vi "Safety_Check.vi"(1 "Adam Loop Count":i32, 2 "Ch Names":string[](array[string]), 3 "Values":dbl[](array[numeric]) format="%.2f") -> (0 "Scan comment":string)   [LabVIEW 2015]
uses:
  ADAM Client/Sub VIs/ADAM Controls/Update_scan_value.ctl
  Anemometry/Anemometry Sub Vis/Globals/Gas_management_global.vi
  ADAM_Global.vi
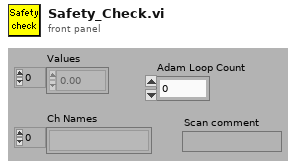
[diagram p1: front panel]
types:
  T1 = cluster{"Channel name":string, "Set value of A to":dbl, "Set value of B to":dbl, "Set value of C to":dbl, "Set value of D to":dbl}
  T2 = typedef "Update_scan_value.ctl" = cluster{"Channel Name":string, "New Value":dbl}
  T3 = enum16{"Append to Global", "Read Global then Clear"}
  T4 = enum16{"On", "Off", "Always On", "Always Off", "Delete"}
  T5 = typedef "LVDateTimeRec.ctl" = cluster{"fractional second":dbl, "second":i32, "minute":i32, "hour":i32, "day of month":i32, "month":i32, "year":i32, "day of week":i32, "day of year":i32, "DST":i32}
  T6 = cluster{"Channel name":string, "Set value of A to":dbl, "Set value of B to":dbl, "Set value of C to":dbl, "Set value of D to":dbl}[]
  T7 = typedef "Ch_description_ADAM.ctl" = cluster{"Ch Name":string, "Type":T8, "Function":T9, "Ch State":T10, "Calibration type":T11, "A":dbl, "B":dbl, "C":dbl, "D":dbl, "Comments":string, "Address":T12, "String":string, "Duty":u16}
  T8 = typedef "Module_type_ADAM.ctl" = string
  T9 = typedef "Function_ADAM.ctl" = enum16{"Analogue Input", "Digital Input", "Event counter", "Event rate", "Analogue Output", "Digital Output", "Relay Output"}
  T10 = typedef "Channel_State.ctl" = enum16{"On", "Off", "Always On", "Always Off"}
  T11 = typedef "Calib_type_ADAM.ctl" = enum16{"Raw", "Bx + A", "Cx^2 + Bx + A", "Dx^3 + Cx^2 + Bx + A", "In Band", "Hi-Tec Q", "Hi-Tec M_dot", "Text"}
  T12 = typedef "Address.ctl" = cluster{"Main":i32, "Ch.":i32, "Sub":i32, "Port Name":string}
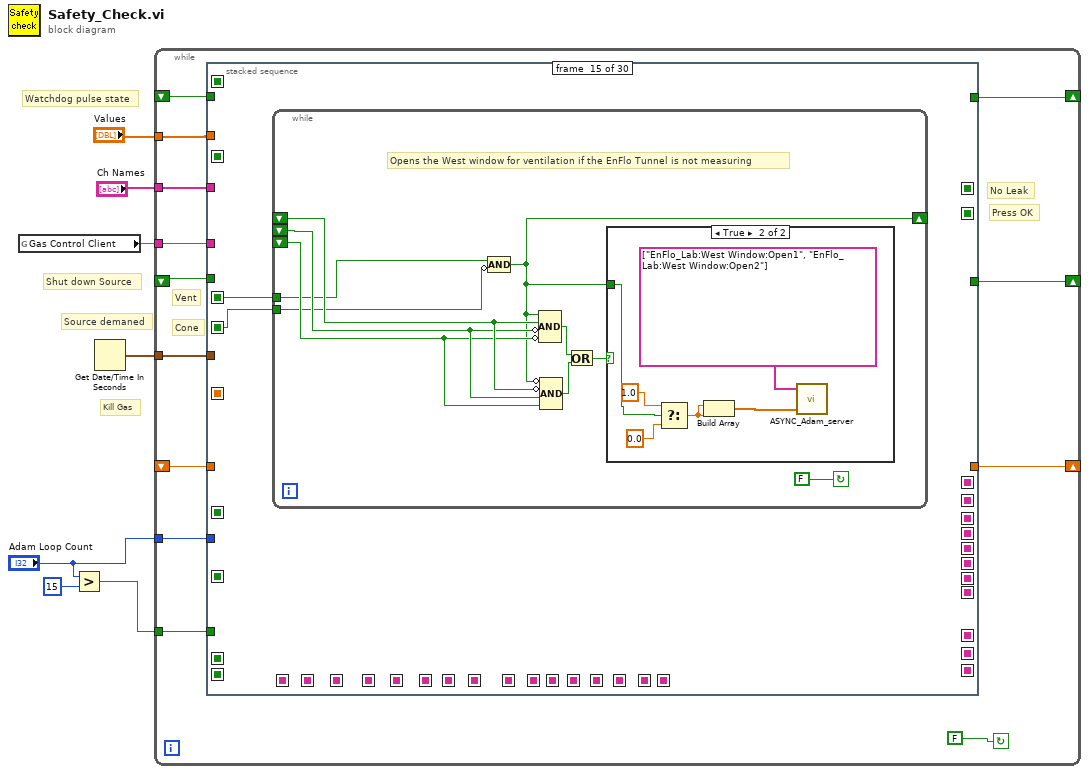
[diagram p0: block diagram]
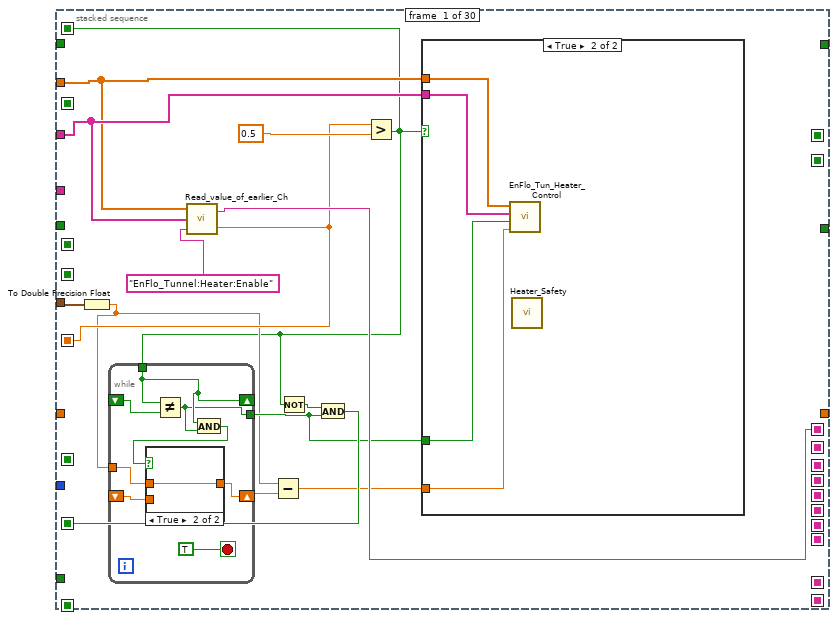
[diagram p2: hidden frame]
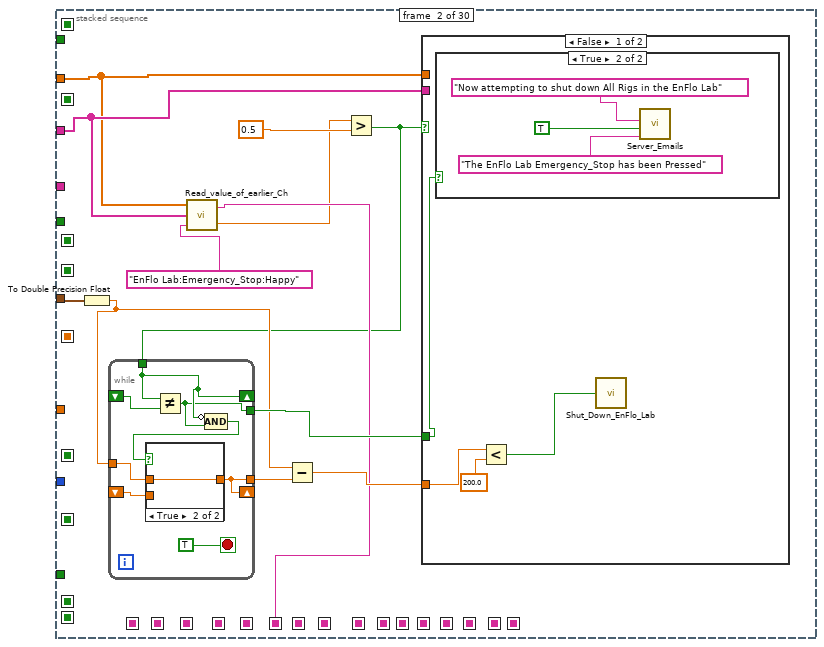
[diagram p5: hidden frame]
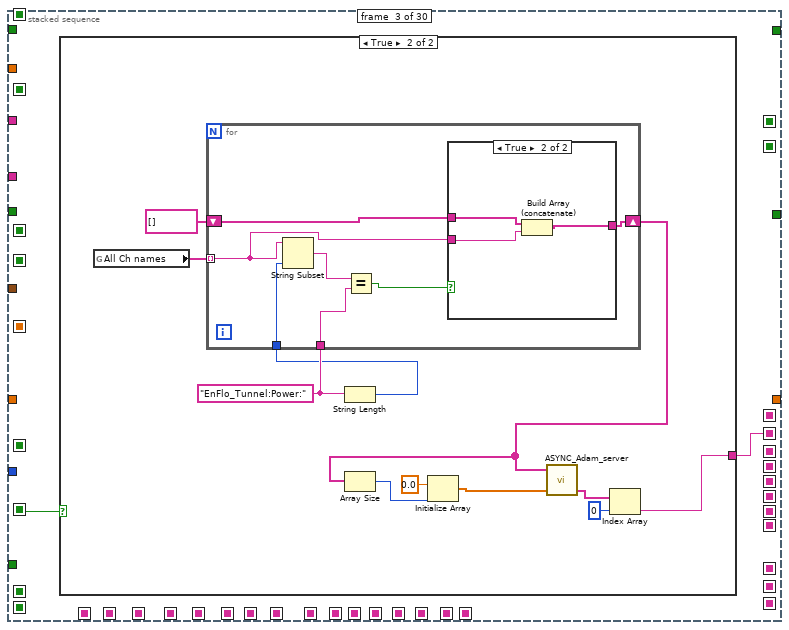
[diagram p9: hidden frame]
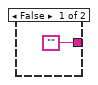
[diagram p10: hidden frame]
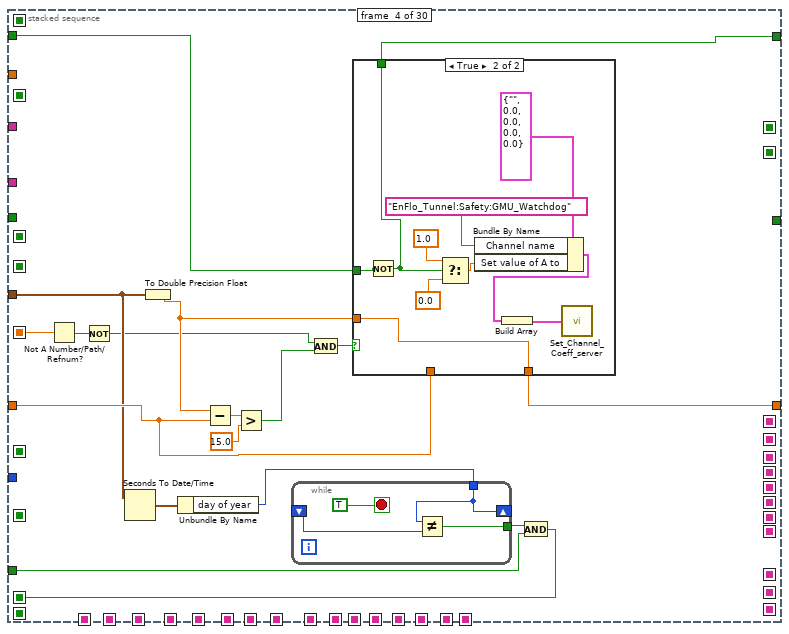
[diagram p12: hidden frame]
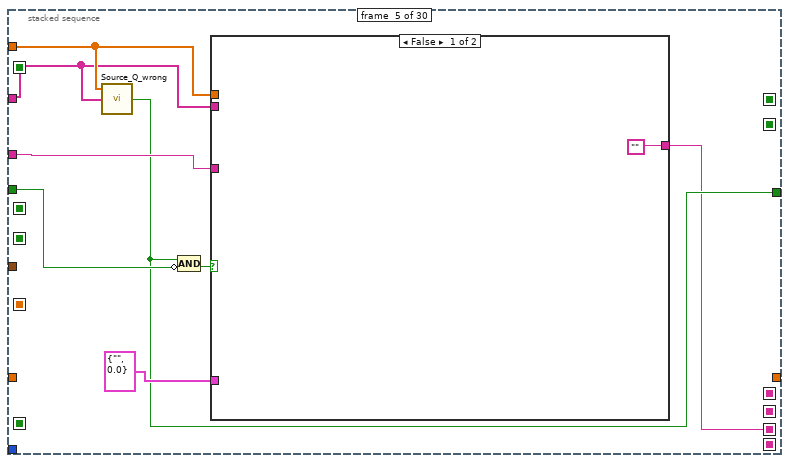
[diagram p14: hidden frame]
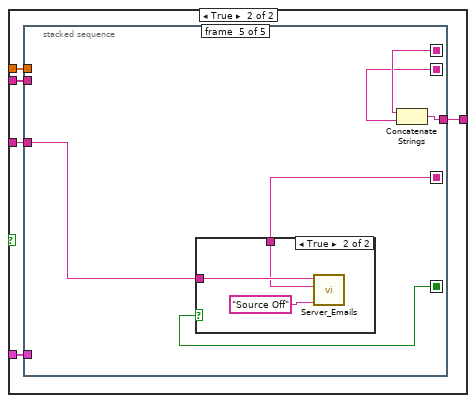
[diagram p15: hidden frame]
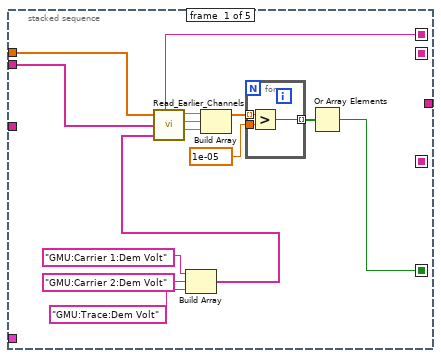
[diagram p16: hidden frame]
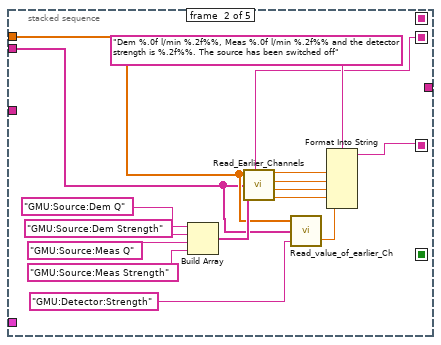
[diagram p17: hidden frame]
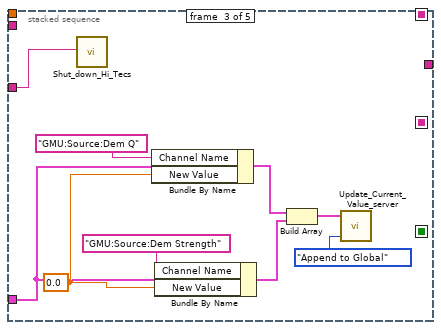
[diagram p18: hidden frame]
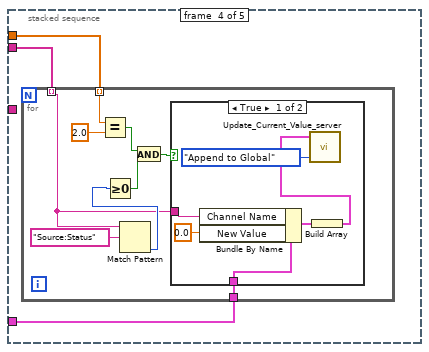
[diagram p19: hidden frame]
diagram:
  # "Shut down Source"
  # "Source demaned"
  # "Watchdog pulse state"
  # "Kill Gas"
  n1 = global read "Gas_management_global.vi" "Gas Control Client"() -> (w5:string)
  n2 = Greater?(x="Adam Loop Count", y=15) -> (0:w3:bool)
  n3 = Get Date/Time In Seconds() -> (seconds since 1Jan1904=w2:timestamp)
  n4 = while {
    shift-left: _ -> [w15]
    shift-right: [w14] -> _
    shift-left: _ -> [w17]
    shift-right: [w16] -> _
    tunnel: w5 -> [w19]
    tunnel: "Ch Names" -> [w20]
    tunnel: "Values" -> [w18]
    shift-right: [w12] -> _
    shift-left: _ -> [w11]
    tunnel: w3 -> [w10]
    tunnel: w2 -> [w9]
    tunnel: "Adam Loop Count" -> [w8]
    stop <- FALSE continue-if-true
    # "Cone"
    # "Vent"
    # "Press OK"
    # "No Leak"
    n5 = stacked-sequence {
      seq-local: [_ _ _ _ _ _ _ w260 _ _ _ _ _ _ _ _ _ _ _ _ _ _ _ _ _ _ _ _ _ _] -> [_ _ _ _ _ _ _ _ _ _ _ _ _ _ _ _ _ _ _ w623 _ _ _ _ _ _ _ _ _ _]
      seq-local: [w28 _ _ _ _ _ _ _ _ _ _ _ _ _ _ _ _ _ _ _ _ _ _ _ _ _ _ _ _ _] -> [_ _ w79 _ _ _ _ _ _ _ _ _ _ _ _ _ _ _ _ _ _ _ _ _ _ _ _ _ _ _]
      seq-local: [_ _ _ w109 _ _ _ _ _ _ _ _ _ _ _ _ _ _ _ _ _ _ _ _ _ _ _ _ _ _] -> [_ _ _ _ _ _ _ _ _ _ _ _ _ _ _ _ _ _ _ _ _ _ _ _ _ _ _ _ _ _]
      seq-local: [_ _ _ _ _ _ _ _ _ _ _ _ _ _ _ _ _ _ _ _ _ _ _ w753 _ _ _ _ _ _] -> [_ _ _ _ _ _ _ _ _ _ _ _ _ _ _ _ _ _ _ _ _ _ _ _ w765 _ _ _ _ _]
      seq-local: [_ _ _ _ _ _ _ _ _ _ _ _ _ _ _ _ _ _ _ _ _ _ _ _ w760 _ _ _ _ _] -> [_ _ _ _ _ _ _ _ _ _ _ _ _ _ _ _ _ _ _ _ _ _ _ _ _ _ _ w874 _ _]
      seq-local: [w30 _ _ _ _ _ _ _ _ _ _ _ _ _ _ _ _ _ _ _ _ _ _ _ _ _ _ _ _ _] -> [_ _ _ _ _ _ _ _ _ _ _ _ _ _ _ _ _ _ _ _ _ _ _ _ _ _ _ _ _ w957]
      seq-local: [_ _ w78 _ _ _ _ _ _ _ _ _ _ _ _ _ _ _ _ _ _ _ _ _ _ _ _ _ _ _] -> [_ _ _ _ _ _ _ _ _ _ _ _ _ _ _ _ _ _ _ _ _ _ _ _ _ _ _ _ _ w956]
      seq-local: [_ _ _ _ w137 _ _ _ _ _ _ _ _ _ _ _ _ _ _ _ _ _ _ _ _ _ _ _ _ _] -> [_ _ _ _ _ _ _ _ _ _ _ _ _ _ _ _ _ _ _ _ _ _ _ _ _ _ _ _ _ w955]
      seq-local: [_ _ _ _ _ w220 _ _ _ _ _ _ _ _ _ _ _ _ _ _ _ _ _ _ _ _ _ _ _ _] -> [_ _ _ _ _ _ _ _ _ _ _ _ _ _ _ _ _ _ _ _ _ _ _ _ _ _ _ _ _ w954]
      seq-local: [_ _ _ _ _ _ w240 _ _ _ _ _ _ _ _ _ _ _ _ _ _ _ _ _ _ _ _ _ _ _] -> [_ _ _ _ _ _ _ _ _ _ _ _ _ _ _ _ _ _ _ _ _ _ _ _ _ _ _ _ _ w953]
      seq-local: [_ _ _ _ _ _ _ w259 _ _ _ _ _ _ _ _ _ _ _ _ _ _ _ _ _ _ _ _ _ _] -> [_ _ _ _ _ _ _ _ _ _ _ _ _ _ _ _ _ _ _ _ _ _ _ _ _ _ _ _ _ w952]
      seq-local: [_ _ _ _ _ _ _ _ _ _ w371 _ _ _ _ _ _ _ _ _ _ _ _ _ _ _ _ _ _ _] -> [_ _ _ _ _ _ _ _ _ _ _ _ _ _ _ _ _ _ _ _ _ _ _ _ _ _ _ _ _ w951]
      seq-local: [_ _ _ _ _ _ _ _ _ _ _ w403 _ _ _ _ _ _ _ _ _ _ _ _ _ _ _ _ _ _] -> [_ _ _ _ _ _ _ _ _ _ _ _ _ _ _ _ _ _ _ _ _ _ _ _ _ _ _ _ _ w942]
      seq-local: [_ _ _ _ _ _ _ _ _ _ _ _ _ _ _ _ w549 _ _ _ _ _ _ _ _ _ _ _ _ _] -> [_ _ _ _ _ _ _ _ _ _ _ _ _ _ _ _ _ _ _ _ _ _ _ _ _ _ _ _ _ w941]
      seq-local: [_ _ _ _ _ _ _ _ _ _ _ _ _ _ _ _ _ _ _ w624 _ _ _ _ _ _ _ _ _ _] -> [_ _ _ _ _ _ _ _ _ _ _ _ _ _ _ _ _ _ _ _ _ _ _ _ _ _ _ _ _ w944]
      seq-local: [_ _ _ _ _ _ _ _ _ _ _ _ _ _ _ _ _ _ _ _ w652 _ _ _ _ _ _ _ _ _] -> [_ _ _ _ _ _ _ _ _ _ _ _ _ _ _ _ _ _ _ _ _ _ _ _ _ _ _ _ _ w945]
      seq-local: [_ _ _ _ _ _ _ _ _ _ _ _ _ _ _ _ _ _ _ _ _ _ _ w747 _ _ _ _ _ _] -> [_ _ _ _ _ _ _ _ _ _ _ _ _ _ _ _ _ _ _ _ _ _ _ _ _ _ _ _ _ w946]
      seq-local: [_ _ _ _ _ _ _ _ _ _ _ _ _ _ _ _ _ _ _ _ _ _ _ _ w757 _ _ _ _ _] -> [_ _ _ _ _ _ _ _ _ _ _ _ _ _ _ _ _ _ _ _ _ _ _ _ _ _ _ _ _ w947]
      seq-local: [_ _ _ _ _ _ _ _ _ _ _ _ w434 _ _ _ _ _ _ _ _ _ _ _ _ _ _ _ _ _] -> [_ _ _ _ _ _ _ _ _ _ _ _ _ _ _ _ _ _ _ _ _ _ _ _ _ _ _ _ _ w948]
      seq-local: [_ _ _ _ _ _ _ _ _ _ _ _ _ _ _ _ _ _ _ _ _ _ _ _ _ _ w836 _ _ _] -> [_ _ _ _ _ _ _ _ _ _ _ _ _ _ _ _ _ _ _ _ _ _ _ _ _ _ _ _ _ w949]
      seq-local: [_ _ _ _ _ _ _ _ _ _ _ _ _ _ _ _ _ _ _ _ _ _ _ _ _ _ _ w872 _ _] -> [_ _ _ _ _ _ _ _ _ _ _ _ _ _ _ _ _ _ _ _ _ _ _ _ _ _ _ _ _ w950]
      seq-local: [w29 _ _ _ _ _ _ _ _ _ _ _ _ _ _ _ _ _ _ _ _ _ _ _ _ _ _ _ _ _] -> [_ _ _ w107 _ _ _ _ _ _ _ _ _ _ _ _ _ _ _ _ _ _ _ _ _ _ _ _ _ _]
      seq-local: [_ _ _ _ _ _ _ _ w278 _ _ _ _ _ _ _ _ _ _ _ _ _ _ _ _ _ _ _ _ _] -> [_ _ _ _ _ _ _ _ _ _ _ _ _ _ _ _ _ _ _ w622 _ _ _ _ _ _ _ _ _ _]
      seq-local: [_ _ _ _ _ _ _ _ w277 _ _ _ _ _ _ _ _ _ _ _ _ _ _ _ _ _ _ _ _ _] -> [_ _ _ _ _ _ _ _ _ _ _ _ _ _ _ _ _ _ _ _ _ _ _ _ _ _ _ _ _ w940]
      seq-local: [_ _ _ _ _ _ _ _ w276 _ _ _ _ _ _ _ _ _ _ _ _ _ _ _ _ _ _ _ _ _] -> [_ _ _ _ _ _ _ _ _ w308 _ _ _ _ _ _ _ _ _ _ _ _ _ w748 w756 w821 _ _ _ _]
      seq-local: [_ _ _ _ _ _ _ _ _ w305 _ _ _ _ _ _ _ _ _ _ _ _ _ _ _ _ _ _ _ _] -> [_ _ _ _ _ _ _ _ _ _ _ _ _ _ _ _ _ _ _ _ _ _ _ _ _ _ _ _ _ w938]
      seq-local: [_ _ _ _ _ _ _ _ _ _ _ _ _ _ _ w503 _ _ _ _ _ _ _ _ _ _ _ _ _ _] -> [_ _ _ _ _ _ _ _ _ _ _ _ _ _ _ _ _ _ _ _ _ _ _ _ _ _ _ _ _ w939]
      seq-local: [_ _ _ _ _ _ _ _ _ _ _ _ _ _ _ _ _ _ _ _ _ _ w715 _ _ _ _ _ _ _] -> [_ _ _ _ _ _ _ _ _ _ _ _ _ _ _ _ _ _ _ _ _ _ _ _ _ _ _ _ _ w937]
      seq-local: [_ _ _ _ _ _ _ _ _ _ _ _ _ w462 _ _ _ _ _ _ _ _ _ _ _ _ _ _ _ _] -> [_ _ _ _ _ _ _ _ _ _ _ _ _ _ _ _ _ _ _ _ _ _ _ _ _ _ _ _ _ w936]
      seq-local: [_ w52 _ _ _ _ _ _ _ _ _ _ _ _ _ _ _ _ _ _ _ _ _ _ _ _ _ _ _ _] -> [_ _ _ _ _ _ _ _ _ _ _ _ _ _ _ _ _ _ _ _ _ _ _ _ _ _ _ _ _ w935]
      seq-local: [_ _ _ _ _ _ _ _ _ _ _ _ _ _ _ _ _ _ _ _ _ _ _ _ _ _ _ _ w894 _] -> [_ _ _ _ _ _ _ _ _ _ _ _ _ _ _ _ _ _ _ _ _ _ _ _ _ _ _ _ _ w934]
      seq-local: [_ _ _ _ _ _ _ _ _ _ _ _ _ _ _ _ _ w570 _ _ _ _ _ _ _ _ _ _ _ _] -> [_ _ _ _ _ _ _ _ _ _ _ _ _ _ _ _ _ _ _ _ _ _ _ _ _ _ _ _ _ w932]
      seq-local: [_ _ _ _ _ _ _ _ _ _ _ _ _ _ _ _ _ _ w602 _ _ _ _ _ _ _ _ _ _ _] -> [_ _ _ _ _ _ _ _ _ _ _ _ _ _ _ _ _ _ _ _ _ _ _ _ _ _ _ _ _ w933]
      seq-local: [w21 _ _ _ _ _ _ _ _ _ _ _ _ _ _ _ _ _ _ _ _ _ _ _ _ _ _ _ _ _] -> [_ _ _ _ _ _ _ _ _ _ _ _ _ _ _ _ _ _ _ _ w651 w672 _ _ _ _ _ _ _ _]
      seq-local: [_ _ _ _ _ _ _ _ _ _ _ _ _ _ _ _ _ _ _ _ _ w670 _ _ _ _ _ _ _ _] -> [_ _ _ _ _ _ _ _ _ _ _ _ _ _ _ _ _ _ _ _ _ _ _ _ _ _ _ _ _ w931]
      seq-local: [_ _ _ _ _ _ _ _ _ _ _ _ _ _ _ _ _ _ _ _ _ _ _ _ _ w820 _ _ _ _] -> [_ _ _ _ _ _ _ _ _ _ _ _ _ _ _ _ _ _ _ _ _ _ _ _ _ _ _ _ _ w930]
      seq-local: [_ _ _ _ _ _ _ _ _ _ _ _ w423 _ _ _ _ _ _ _ _ _ _ _ _ _ _ _ _ _] -> [_ _ _ _ _ _ _ _ _ _ _ _ _ _ w483 _ _ _ _ _ _ _ _ _ _ _ _ _ _ _]
      seq-local: [_ _ _ _ _ _ _ _ _ _ _ _ _ w461 _ _ _ _ _ _ _ _ _ _ _ _ _ _ _ _] -> [_ _ _ _ _ _ _ _ _ _ _ _ _ _ w484 _ _ _ _ _ _ _ _ _ _ _ _ _ _ _]
      tunnel: w20 -> [w32 w58 _ _ w139 w227 w242 w261 w279 w306 w372 w404 w433 w463 _ w504 w551 w572 w604 w625 w656 w676 w709 w751 w766 _ w839 _ _ _]
      tunnel: w19 -> [_ _ _ _ w144 _ w241 _ _ _ _ _ _ _ _ _ _ _ _ _ _ _ _ _ _ _ _ _ _ _]
      tunnel: w18 -> [w31 w57 _ _ w140 w223 w243 w262 w280 w307 w373 w405 w431 w464 _ w505 w552 w573 w605 w626 w657 w677 w708 w752 w767 _ w840 _ _ _]
      tunnel: w17 -> [_ _ _ w120 _ _ _ _ _ _ _ _ _ _ _ _ _ _ _ _ _ _ _ _ _ _ _ _ _ _]
      tunnel: [_ _ _ w119 _ _ _ _ _ _ _ _ _ _ _ _ _ _ _ _ _ _ _ _ _ _ _ _ _ _] -> w16
      tunnel: w15 -> [_ _ _ _ w143 _ _ _ _ _ _ _ _ _ _ _ _ _ _ _ _ _ _ _ _ _ _ _ _ _]
      tunnel: [_ _ _ _ w138 _ _ _ _ _ _ _ _ _ _ _ _ _ _ _ _ _ _ _ _ _ _ _ _ _] -> w14
      tunnel: [_ _ _ w118 _ _ _ _ _ _ _ _ _ _ _ _ _ _ _ _ _ _ _ _ _ _ _ _ _ _] -> w12
      tunnel: w11 -> [_ _ _ w114 _ _ _ _ _ _ _ _ _ _ _ _ _ _ _ _ _ _ _ _ _ _ _ _ _ _]
      tunnel: w10 -> [_ _ _ w110 _ _ _ _ _ _ _ _ w435 _ _ w501 w550 w571 w603 _ _ _ _ _ w761 w819 _ w873 _ _]
      tunnel: w9 -> [w25 w55 _ w108 _ _ _ _ _ _ _ _ _ _ _ w502 _ _ _ _ _ _ _ _ _ _ _ _ _ _]
      tunnel: w8 -> [_ _ _ _ _ _ _ _ _ _ _ _ _ _ _ _ _ _ _ _ _ _ _ _ _ _ _ _ w907 _]
      frame #0 {
        n6 = To Double Precision Float(number=w25) -> (double precision float=w24:dbl)
        n7 = call "Read_value_of_earlier_Ch.vi"("Desired Ch to Read"="EnFlo_Tunnel:Heater:Enable", "Ch names"=w32, "Present scan array"=w31) -> ("Value"=w29:dbl, "Scan comment"=w30:string)  [unwired: 1 in]
        n8 = Greater?(x=w29, y=0.5) -> (0:w21:bool)
        n9 = while {
          shift-right: [w40] -> _
          shift-left: _ -> [w42]
          tunnel: w21 -> [w40]
          tunnel: [w39] -> w26
          shift-right: [w37] -> w23
          shift-left: _ -> [w35]
          tunnel: w24 -> [w36]
          stop <- TRUE stop-if-true
          n10 = Not Equal?(x=w40, y=w42) -> (x != y?=w39:bool)
          n11 = And(x=w40, y=w39) -> (x .and. y?=w38:bool)
          n12 = case shown="True" w38 {
            tunnel: [w43 w44] -> w37
            tunnel: w36 -> [_ w44]
            tunnel: w35 -> [w43 _]
            frame False {
            }
            frame True {
            }
          }
        }
        n13 = Subtract(x=w24, y=w23) -> (x-y=w22:dbl)
        n14 = Not(x=w21) -> (.not. x?=w27:bool)
        n15 = And(x=w27, y=w26) -> (x .and. y?=w28:bool)
        n16 = case shown="True" w21 {
          tunnel: w31 -> [_ w48]
          tunnel: w32 -> [_ w47]
          tunnel: w26 -> [_ w46]
          tunnel: w22 -> [_ w45]
          frame False {
          }
          frame True {
            n17 = call "EnFlo_Tun_Heater_Control.vi"("Heaters Enabled time (s)"=w45, "Heaters Just Enabled"=w46, "Ch Names"=w47, "Values"=w48) -> ()  [unwired: 1 in]
            n18 = call "Heater_Safety.vi"() -> ()  [unwired: 3 in, 5 out]
          }
        }
      }
      frame #1 {
        n19 = To Double Precision Float(number=w55) -> (double precision float=w54:dbl)
        n20 = call "Read_value_of_earlier_Ch.vi"("Desired Ch to Read"="EnFlo Lab:Emergency_Stop:Happy", "Ch names"=w58, "Present scan array"=w57) -> ("Value"=w50:dbl, "Scan comment"=w52:string)  [unwired: 1 in]
        n21 = Greater?(x=w50, y=0.5) -> (0:w51:bool)
        n22 = while {
          shift-right: [w66] -> _
          shift-left: _ -> [w68]
          tunnel: w51 -> [w66]
          tunnel: [w65] -> w56
          shift-right: [w61] -> _
          shift-left: _ -> [w62]
          tunnel: w54 -> [w63]
          tunnel: [w61] -> w49
          stop <- TRUE stop-if-true
          n23 = Not Equal?(x=w66, y=w68) -> (x != y?=w65:bool)
          n24 = Compound Arithmetic op=AND(invert w66, w65) -> (w64:bool)
          n25 = case shown="True" w64 {
            tunnel: [w69 w70] -> w61
            tunnel: w63 -> [_ w70]
            tunnel: w62 -> [w69 _]
            frame False {
            }
            frame True {
            }
          }
        }
        n26 = Subtract(x=w54, y=w49) -> (x-y=w53:dbl)
        n27 = case shown="False" w51 {
          tunnel: w57 -> [_ _]
          tunnel: w58 -> [_ _]
          tunnel: w56 -> [w72 _]
          tunnel: w53 -> [w74 _]
          frame False {
            n28 = case shown="True" w72 {
              frame False {
              }
              frame True {
                n29 = call "Server_Emails.vi"("Message"="Now attempting to shut down All Rigs in the EnFlo Lab", "Contact All clients?"=TRUE, "Subject"="The EnFlo Lab Emergency_Stop has been Pressed") -> ()  [unwired: 2 in, 3 out]
              }
            }
            n30 = Less?(x=w74, y=200.0) -> (x < y?=w71:bool)
            n31 = call "Shut_Down_EnFlo_Lab.vi"("Initial Shutdown"=w71) -> ()
          }
          frame True {
          }
        }
      }
      frame #2 {
        n32 = case shown="True" w79 {
          tunnel: ["" w82] -> w78
          frame False {
          }
          frame True {
            w91 = "EnFlo_Tunnel:Power:"
            n33 = global read "ADAM_Global.vi" "All Ch names"() -> (w81:string[])
            n34 = String Length(string=w91) -> (length=w90:i32)
            n35 = for {
              shift-right: [w93] -> w86
              shift-left: string[] [] -> [w94]
              tunnel: w81 -> [w97] mode=indexing
              tunnel: w90 -> [w98]
              tunnel: w91 -> [w95]
              n36 = String Subset(string=w97, length (rest)=w98) -> (substring=w96:string)  [unwired: 1 out]
              n37 = Equal?(x=w96, y=w95) -> (x = y?=w92:bool)
              n38 = case shown="True" w92 {
                tunnel: w97 -> [_ w102]
                tunnel: w94 -> [w99 w100]
                tunnel: [w99 w101] -> w93
                frame False {
                }
                frame True {
                  n39 = Build Array (concatenate)(w100, w102) -> (w101:string[])
                }
              }
            }
            n40 = Array Size(array=w86) -> (size(s)=w87:i32)
            n41 = Initialize Array(0.0 ("element"), w87) -> (w85:dbl[])
            n42 = call "ASYNC_Adam_server.vi"("Values"=w85, "Channel Names"=w86) -> ("Scan Comments"=w84:string[])  [unwired: 1 in, 2 out]
            n43 = Index Array(array=w84, index=0) -> (element=w82:string)
          }
        }
      }
      frame #3 {
        n44 = Not A Number/Path/Refnum?(number/path/refnum=w107) -> (NaN/Path/Refnum?=w106:bool)
        n45 = Not(x=w106) -> (.not. x?=w104:bool)
        n46 = Seconds To Date/Time(time stamp (now)=w108) -> (date time rec=w113:T5)  [unwired: 1 in]
        n47 = To Double Precision Float(number=w108) -> (double precision float=w117:dbl)
        n48 = Unbundle By Name(w113) -> ("day of year"=w112:i32)
        n49 = Subtract(x=w117, y=w114) -> (x-y=w116:dbl)
        n50 = Greater?(x=w116, y=15.0) -> (0:w105:bool)
        n51 = while {
          shift-right: [w124] -> _
          shift-left: _ -> [w123]
          tunnel: w112 -> [w124]
          tunnel: [w122] -> w111
          stop <- TRUE stop-if-true
          n52 = Not Equal?(x=w124, y=w123) -> (x != y?=w122:bool)
        }
        n53 = And(x=w104, y=w105) -> (x .and. y?=w103:bool)
        n54 = case shown="True" w103 {
          tunnel: w120 -> [w125 w129]
          tunnel: [w125 w128] -> w119
          tunnel: [w126 w127] -> w118
          tunnel: w117 -> [_ w127]
          tunnel: w114 -> [w126 _]
          frame False {
          }
          frame True {
            n55 = Not(x=w129) -> (.not. x?=w128:bool)
            n56 = Select(t=1.0 ("Suction"), s=w128, f=0.0 ("Suction")) -> (s? t:f=w132:dbl)
            n57 = Bundle By Name(cluster=T1 {"Channel name"="", "Set value of A to"=0.0, "Set value of B to"=0.0, "Set value of C to"=0.0, "Set value of D to"=0.0}, "Channel name"="EnFlo_Tunnel:Safety:GMU_Watchdog" ("Desired Ch to Read"), "Set value of A to"=w132) -> (w136:T1)
            n58 = Build Array(w136) -> (w131:T6)
            n59 = call "Set_Channel_Coeff_server.vi"("Set Array"=w131) -> ()
          }
        }
        n60 = And(x=w111, y=w110) -> (x .and. y?=w109:bool)
      }
      frame #4 {
        n61 = call "Source_Q_wrong.vi"("Ch Names"=w139, "Values"=w140) -> ("Gas Error?"=w138:bool)  [unwired: 1 out]
        n62 = Compound Arithmetic op=AND(w138, invert w143) -> (w142:bool)
        n63 = case shown="False" w142 {
          tunnel: w144 -> [_ w150]
          tunnel: w140 -> [_ w149]
          tunnel: w139 -> [_ w148]
          tunnel: T2 {"Channel Name"="", "New Value"=0.0} ("Update Scan Value Cluster") -> [_ w147]
          tunnel: ["" w146] -> w137
          frame False {
          }
          frame True {
            n64 = stacked-sequence {
              seq-local: [_ w182 _ _ _] -> [_ _ _ _ w215]
              seq-local: [w152 _ _ _ _] -> [_ _ _ _ w214]
              seq-local: [w151 _ _ _ _] -> [_ _ _ _ w213]
              seq-local: [_ w168 _ _ _] -> [_ _ _ _ w212]
              tunnel: w150 -> [_ _ w185 _ w216]
              tunnel: w149 -> [w162 w172 _ w194 _]
              tunnel: w148 -> [w163 w171 _ w195 _]
              tunnel: w147 -> [_ _ w184 w193 _]
              tunnel: [_ _ _ _ w211] -> w146
              frame #0 {
                n65 = Build Array("GMU:Carrier 1:Dem Volt", "GMU:Carrier 2:Dem Volt", "GMU:Trace:Dem Volt") -> (w164:string[])
                n66 = call "Read_Earlier_Channels.vi"("Present scan array"=w162, "Ch names"=w163, "Desired Channels"=w164) -> ("Scan comments"=w151:string, "Index 0"=w158:dbl, "Index 1"=w157:dbl, "Index 2"=w156:dbl)  [unwired: 2 out]
                n67 = Build Array(w158, w157, w156) -> (w155:dbl[])
                n68 = for {
                  tunnel: w155 -> [w167] mode=indexing
                  tunnel: 1e-05 -> [w166]
                  tunnel: [w165] -> w153 mode=indexing
                  n69 = Greater?(x=w167, y=w166) -> (0:w165:bool)
                }
                n70 = Or Array Elements(Boolean array=w153) -> (logical OR=w152:bool)
              }
              frame #1 {
                n71 = Build Array("GMU:Source:Dem Q", "GMU:Source:Dem Strength", "GMU:Source:Meas Q", "GMU:Source:Meas Strength") -> (w177:string[])
                n72 = call "Read_Earlier_Channels.vi"("Present scan array"=w172, "Ch names"=w171, "Desired Channels"=w177) -> ("Scan comments"=w168:string, "Index 0"=w176:dbl, "Index 1"=w175:dbl, "Index 2"=w174:dbl, "Index 3"=w173:dbl)  [unwired: 1 out]
                n73 = call "Read_value_of_earlier_Ch.vi"("Desired Ch to Read"="GMU:Detector:Strength", "Ch names"=w171, "Present scan array"=w172) -> ("Value"=w169:dbl)  [unwired: 1 in, 1 out]
                n74 = Format Into String(format string="Dem %.0f l/min %.2f%%, Meas %.0f l/min %.2f%% and the detector strength is %.2f%%. The source has been switched off" ("Format String"), w176, w175, w174, w173, w169) -> (resulting string=w182:string)  [unwired: 2 in, 1 out]
              }
              frame #2 {
                w186 = 0.0 ("Bundle Element")
                n75 = call "Shut_down_Hi_Tecs.vi"("Client Name"=w185) -> ()  [unwired: 6 out]
                n76 = Bundle By Name(cluster=w184, "Channel Name"="GMU:Source:Dem Q", "New Value"=w186) -> (w191:T2)
                n77 = Bundle By Name(cluster=w184, "Channel Name"="GMU:Source:Dem Strength", "New Value"=w186) -> (w192:T2)
                n78 = Build Array(w191, w192) -> (w188:T2[])
                n79 = call "Update_Current_Value_server.vi"("Mode"=T3."Append to Global", "Update array in"=w188) -> ()  [unwired: 1 in, 1 out]
              }
              frame #3 {
                n80 = for {
                  tunnel: w195 -> [w196] mode=indexing
                  tunnel: w194 -> [w202] mode=indexing
                  tunnel: w193 -> [w197]
                  n81 = Equal?(x=w202, y=2.0) -> (x = y?=w199:bool)
                  n82 = Match Pattern(string=w196, regular expression="Source:Status") -> (offset past match=w203:i32)  [unwired: 4 out]
                  n83 = Greater Or Equal To 0?(x=w203) -> (x >= 0?=w200:bool)
                  n84 = And(x=w199, y=w200) -> (x .and. y?=w198:bool)
                  n85 = case shown="True" w198 {
                    tunnel: w197 -> [w210 _]
                    tunnel: w196 -> [w209 _]
                    frame True {
                      n86 = Bundle By Name(cluster=w210, "Channel Name"=w209, "New Value"=0.0) -> (w207:T2)
                      n87 = Build Array(w207) -> (w206:T2[])
                      n88 = call "Update_Current_Value_server.vi"("Mode"=T3."Append to Global", "Update array in"=w206) -> ()  [unwired: 1 in, 1 out]
                    }
                    frame False {
                    }
                  }
                }
              }
              frame #4 {
                n89 = case shown="True" w214 {
                  tunnel: w216 -> [_ w219]
                  tunnel: w215 -> [_ w218]
                  frame False {
                  }
                  frame True {
                    n90 = call "Server_Emails.vi"("Client Name Contains"=w219, "Message"=w218, "Subject"="Source Off") -> ()  [unwired: 2 in, 3 out]
                  }
                }
                n91 = Concatenate Strings(w213, w212) -> (w211:string)
              }
            }
          }
        }
      }
      frame #5 {
        n92 = global read "ADAM_Global.vi" "Program Hung Clients"() -> (w228:string[])
        n93 = for {
          tunnel: w228 -> [w237] mode=indexing
          tunnel: w223 -> [w239]
          tunnel: w227 -> [w238]
          tunnel: [w235] -> w226 mode=indexing
          tunnel: [w232] -> w225 mode=indexing
          shift-right: [w230] -> w220
          shift-left: "" -> [w231]
          n94 = call "Split_Ch_name.vi"("Ch name"=w237) -> ("Low level"=w234:string)  [unwired: 2 out]
          n95 = call "Shut_Down_Client_Demands.vi"("Ch Names"=w238, "Values"=w239, "Client Name"=w237) -> ("Comments"=w229:string)
          n96 = Concatenate Strings(w231, w229) -> (w230:string)
          n97 = Concatenate Strings(w234, ":Source:Status") -> (w235:string)
          n98 = Concatenate Strings(w234, ":Program:Sync") -> (w232:string)
        }
        n99 = Build Array (concatenate)(w226, w225) -> (w224:string[])
        n100 = call "Cntrl_Ch_Status_low.vi"("Mode"=T4."Delete", "Channel names"=w224) -> ()  [unwired: 1 out]
      }
      frame #6 {
        n101 = while {
          tunnel: w243 -> [w255]
          tunnel: w242 -> [w254]
          shift-right: [w249] -> _
          shift-left: _ -> [w250]
          tunnel: w241 -> [w247]
          tunnel: [w245] -> w240
          stop <- FALSE continue-if-true
          n102 = call "Read_value_of_earlier_Ch.vi"("Desired Ch to Read"="GMU:Detector:Happy", "Ch names"=w254, "Present scan array"=w255) -> ("Value"=w252:dbl, "Scan comment"=w245:string)  [unwired: 1 in]
          n103 = Greater?(x=w252, y=0.5) -> (0:w249:bool)
          n104 = Compound Arithmetic op=AND(invert w249, w250) -> (w248:bool)
          n105 = case shown="True" w248 {
            tunnel: w247 -> [_ w257]
            frame False {
            }
            frame True {
              n106 = call "Server_Emails.vi"("Client Name Contains"=w257, "Message"="The GMU Gas detector IR2100 is unhappy. Please check concentrations etc. This will have turned off the gases from the outside bottle store.  You will need to repress the blue gas button after clearing the fault by purging the source with carrier gas only.", "Subject"="GMU Gas Detector Unhappy") -> ()  [unwired: 2 in, 3 out]
            }
          }
        }
        n107 = global write "ADAM_Global.vi" "Program Hung Clients"(string[] [] ("Program Hung Clients")) -> ()
      }
      frame #7 {
        n108 = while {
          tunnel: w262 -> [w272]
          tunnel: w261 -> [w271]
          shift-right: [w266] -> w260
          shift-left: _ -> [w267]
          tunnel: [w263] -> w259
          stop <- FALSE continue-if-true
          n109 = call "Read_value_of_earlier_Ch.vi"("Desired Ch to Read"="EnFlo Lab:Leak_Detector:Happy", "Ch names"=w271, "Present scan array"=w272) -> ("Value"=w269:dbl, "Scan comment"=w263:string)  [unwired: 1 in]
          n110 = Greater?(x=w269, y=0.5) -> (0:w266:bool)
          n111 = Compound Arithmetic op=AND(invert w266, w267) -> (w265:bool)
          n112 = case shown="True" w265 {
            frame False {
            }
            frame True {
              n113 = call "Server_Emails.vi"("Client Name Contains"="EnFlo_Tunnel", "Message"="The leak detector is indicating a leak under the Enflo Tunnel. The chiller pumps should automaticaly be turned off and the cooling circuit isolated from the  University Chilled water system. The heaters should also have been disabled.", "Subject"="Leak Detected under EnFlo Tunnel") -> ()  [unwired: 2 in, 3 out]
            }
          }
        }
      }
      frame #8 {
        n114 = while {
          tunnel: w280 -> [w286]
          tunnel: w279 -> [w285]
          shift-right: [w297] -> w278
          shift-left: _ -> [w298]
          tunnel: [w289] -> w277
          tunnel: [w281] -> w276
          stop <- FALSE continue-if-true
          n115 = call "Read_value_of_earlier_Ch.vi"("Desired Ch to Read"="EnFlo_Tunnel:Chiller_Pump:Enable", "Ch names"=w285, "Present scan array"=w286) -> ("Value"=w292:dbl, "Scan comment"=w290:string)  [unwired: 1 in]
          n116 = call "Read_value_of_earlier_Ch.vi"("Desired Ch to Read"="EnFlo_Tunnel:Chilled Water:Pressure_OK", "Ch names"=w285, "Present scan array"=w286) -> ("Value"=w300:dbl, "Scan comment"=w291:string)  [unwired: 1 in]
          n117 = call "Read_value_of_earlier_Ch.vi"("Desired Ch to Read"="EnFlo_Tunnel:Chiller_Pump:Running", "Ch names"=w285, "Present scan array"=w286) -> ("Value"=w283:dbl, "Scan comment"=w282:string)  [unwired: 1 in]
          n118 = Greater?(x=w300, y=0.5) -> (0:w297:bool)
          n119 = Greater?(x=w292, y=0.5) -> (0:w288:bool)
          n120 = Compound Arithmetic op=AND(invert w297, w298, w288) -> (w296:bool)
          n121 = case shown="True" w296 {
            frame False {
            }
            frame True {
              n122 = call "Server_Emails.vi"("Client Name Contains"="EnFlo_Tunnel", "Message"="The pressure in the chilled water  for the Enflo Tunnel has tripped the system. The chiller pumps should automaticaly be turned off and the cooling circuit isolated from the  University Chilled water system. The heaters should also have been disabled.", "Subject"="EnFlo Chilled Water Overpressure Trip") -> ()  [unwired: 2 in, 3 out]
            }
          }
          n123 = Greater?(x=w283, y=0.5) -> (0:w281:bool)
          n124 = Concatenate Strings(w290, w291, w282) -> (w289:string)
        }
      }
      frame #9 {
        n125 = case shown="True" w308 {
          tunnel: w307 -> [_ w335]
          tunnel: w306 -> [_ w334]
          tunnel: ["" w314] -> w305
          frame False {
          }
          frame True {
            w319 = "EnFlo_Tunnel:Chilled Water:Motor_Dem_Voltage"
            # "EnFlo_Tunnel:Chiller_Pump:Running"
            n126 = call "Read_value_of_earlier_Ch.vi"("Desired Ch to Read"="EnFlo_Tunnel:Chilled Water:Pressure_supply (Bar)", "Ch names"=w334, "Present scan array"=w335) -> ("Value"=w311:dbl, "Scan comment"=w318:string)  [unwired: 1 in]
            n127 = call "Read_value_of_earlier_Ch.vi"("Desired Ch to Read"="EnFlo_Tunnel:Chilled Water:Pressure_return (Bar)", "Ch names"=w334, "Present scan array"=w335) -> ("Value"=w330:dbl, "Scan comment"=w317:string)  [unwired: 1 in]
            n128 = call "Read_value_of_earlier_Ch.vi"("Desired Ch to Read"="EnFlo_Tunnel:Chilled Water:Desired_Delta_P", "Ch names"=w334, "Present scan array"=w335) -> ("Value"=w328:dbl, "Scan comment"=w316:string)  [unwired: 1 in]
            n129 = call "Read_value_of_earlier_Ch.vi"("Desired Ch to Read"=w319, "Ch names"=w334, "Present scan array"=w335) -> ("Value"=w323:dbl, "Scan comment"=w315:string)  [unwired: 1 in]
            n130 = Subtract(x=w311, y=w330) -> (x-y=w329:dbl)
            n131 = Subtract(x=w329, y=w328) -> (x-y=w322:dbl)
            n132 = Concatenate Strings(w318, w317, w316, w315) -> (w314:string)
            n133 = In Range and Coerce(upper limit=0.1 ("lower limit"), x=w322, lower limit=-0.1) -> (In Range?=w313:bool)  [unwired: 1 out]
            n134 = Less?(x=w311, y=3.85) -> (x < y?=w310:bool)
            n135 = Less?(x=w311, y=4.0) -> (x < y?=w324:bool)
            n136 = case shown="True" w324 {
              tunnel: w323 -> [w346 w350]
              tunnel: w313 -> [_ w352]
              tunnel: w322 -> [_ w351]
              tunnel: [TRUE w349] -> w321
              tunnel: [w343 w348] -> w320
              tunnel: w310 -> [_ w347]
              frame False {
                n137 = Subtract(x=w346, y=0.2) -> (x-y=w343:dbl)
              }
              frame True {
                n138 = case shown="False" w352 {
                  tunnel: w351 -> [w358 _]
                  tunnel: w350 -> [w357 w369]
                  tunnel: [TRUE FALSE] -> w349
                  tunnel: [w355 w369] -> w348
                  tunnel: w347 -> [w353 _]
                  frame False {
                    n139 = Greater Than 0?(x=w358) -> (x > 0?=w356:bool)
                    n140 = case shown="False" w356 {
                      tunnel: w357 -> [w360 w364]
                      tunnel: [w359 w363] -> w355
                      tunnel: w353 -> [_ w362]
                      frame True {
                        n141 = Subtract(x=w360, y=0.1) -> (x-y=w359:dbl)
                      }
                      frame False {
                        n142 = case shown="False" w362 {
                          tunnel: w364 -> [w365 w367]
                          tunnel: [w365 w366] -> w363
                          frame False {
                          }
                          frame True {
                            n143 = Add(x=w367, y=0.1) -> (x+y=w366:dbl)
                          }
                        }
                      }
                    }
                  }
                  frame True {
                  }
                }
              }
            }
            n144 = case shown="True" w321 {
              tunnel: w320 -> [_ w337]
              tunnel: w319 -> [_ w340]
              frame False {
              }
              frame True {
                n145 = In Range and Coerce(upper limit=10.0, x=w337, lower limit=0.0) -> (coerced(x)=w336:dbl)  [unwired: 1 out]
                n146 = Build Array(w340) -> (w341:string[])
                n147 = Build Array(w336) -> (w342:dbl[])
                n148 = call "ASYNC_Adam_server.vi"("Values"=w342, "Channel Names"=w341) -> ()  [unwired: 1 in, 3 out]
              }
            }
          }
        }
      }
      frame #10 {
        n149 = while {
          tunnel: w373 -> [w389]
          tunnel: w372 -> [w388]
          shift-right: [w382] -> _
          shift-left: _ -> [w378]
          tunnel: [w374] -> w371
          stop <- FALSE continue-if-true
          w380 = 60.0 ("y")
          n150 = Decrement(x=w380) -> (x-1=w381:dbl)
          n151 = Select(t=w381, s=w378, f=w380) -> (s? t:f=w379:dbl)
          n152 = call "Read_value_of_earlier_Ch.vi"("Desired Ch to Read"="EnFlo_Tunnel:Chilled Water:Motor1 Temp", "Ch names"=w388, "Present scan array"=w389) -> ("Value"=w396:dbl, "Scan comment"=w376:string)  [unwired: 1 in]
          n153 = call "Read_value_of_earlier_Ch.vi"("Desired Ch to Read"="EnFlo_Tunnel:Chilled Water:Motor2 Temp", "Ch names"=w388, "Present scan array"=w389) -> ("Value"=w393:dbl, "Scan comment"=w375:string)  [unwired: 1 in]
          n154 = Greater?(x=w396, y=w379) -> (0:w390:bool)
          n155 = Greater?(x=w393, y=w379) -> (0:w391:bool)
          n156 = Or(x=w390, y=w391) -> (x .or. y?=w384:bool)
          n157 = call "Read_value_of_earlier_Ch.vi"("Desired Ch to Read"="EnFlo_Tunnel:Chiller_Pump:Enable", "Ch names"=w388, "Present scan array"=w389) -> ("Value"=w386:dbl, "Scan comment"=w377:string)  [unwired: 1 in]
          n158 = Greater?(x=w386, y=0.5) -> (0:w383:bool)
          n159 = And(x=w383, y=w384) -> (x .and. y?=w382:bool)
          n160 = Compound Arithmetic op=AND(w382, invert w378) -> (w395:bool)
          n161 = case shown="True" w395 {
            tunnel: w380 -> [_ w399]
            frame False {
            }
            frame True {
              n162 = Format Into String(format string="The Chilled Water Motor Temp is greater than %.0f deg C." ("Message"), w399) -> (resulting string=w398:string)  [unwired: 2 in, 1 out]
              n163 = call "Server_Emails.vi"("Client Name Contains"="EnFlo_Tunnel", "Message"=w398, "Subject"="Chilled Water Motor Temp") -> ()  [unwired: 2 in, 3 out]
            }
          }
          n164 = Concatenate Strings(w377, w376, w375) -> (w374:string)
        }
      }
      frame #11 {
        n165 = while {
          tunnel: w405 -> [w419]
          tunnel: w404 -> [w418]
          shift-right: [w407] -> _
          shift-left: _ -> [w413]
          shift-left: _ -> [w412]
          shift-left: _ -> [w411]
          tunnel: [w406] -> w403
          stop <- FALSE continue-if-true
          n166 = call "Read_value_of_earlier_Ch.vi"("Desired Ch to Read"="FFID:System:Enable", "Ch names"=w418, "Present scan array"=w419) -> ("Value"=w414:dbl, "Scan comment"=w406:string)  [unwired: 1 in]
          n167 = Greater?(x=w414, y=0.5) -> (0:w407:bool)
          n168 = Compound Arithmetic op=AND(w407, w413, invert w412, invert w411) -> (w409:bool)
          n169 = Compound Arithmetic op=AND(invert w407, invert w413, w412, w411) -> (w410:bool)
          n170 = Or(x=w409, y=w410) -> (x .or. y?=w408:bool)
          n171 = case shown="True" w408 {
            tunnel: w414 -> [_ w420]
            tunnel: w407 -> [_ _]
            frame False {
            }
            frame True {
              n172 = Build Array(w420) -> (w422:dbl[])
              n173 = call "ASYNC_Adam_server.vi"("Values"=w422, "Channel Names"=string[] ["GMU:Gas:Enable"]) -> ()  [unwired: 1 in, 3 out]
            }
          }
        }
      }
      frame #12 {
        n174 = Search 1D Array(1D array=w433, element="EnFlo_Tunnel:Motor:Enable" ("Desired Ch to Read")) -> (index of element=w430:i32)  [unwired: 1 out]
        n175 = Search 1D Array(1D array=w433, element="Status:of:EnFlo_Tunnel") -> (index of element=w438:i32)  [unwired: 1 out]
        n176 = Index Array(array=w431, index=w438) -> (element=w429:dbl)
        n177 = Index Array(array=w431, index=w430) -> (element=w428:dbl)
        n178 = To Long Integer(number=w429) -> (32bit integer=w424:i32)
        n179 = Greater?(x=w428, y=0.5) -> (0:w426:bool)
        n180 = case shown="0, Default" w424 {
          tunnel: [FALSE TRUE TRUE TRUE] -> w425
          frame 0, Default {
          }
          frame 1 {
          }
          frame 2 {
          }
          frame 3 {
          }
        }
        n181 = And(x=w425, y=w426) -> (x .and. y?=w423:bool)
        n182 = while {
          shift-right: [w450] -> _
          shift-left: _ -> [w451]
          tunnel: w423 -> [w450]
          tunnel: "EnFlo_Tunnel:Warning_Cone:Enable" -> [w452]
          tunnel: w435 -> [w447]
          tunnel: [w445] -> w434
          stop <- TRUE stop-if-true
          n183 = Not Equal?(x=w450, y=w451) -> (x != y?=w448:bool)
          n184 = Boolean To (0,1)(Boolean=w450) -> (0, 1=w444:i16)
          n185 = To Double Precision Float(number=w444) -> (double precision float=w443:dbl)
          n186 = Compound Arithmetic op=OR(w448, invert w447) -> (w446:bool)
          n187 = Build Array(w452) -> (w453:string[])
          n188 = Build Array(w443) -> (w454:dbl[])
          n189 = case shown="True" w446 {
            tunnel: w454 -> [_ w460]
            tunnel: w453 -> [_ w459]
            tunnel: ["" w456] -> w445
            frame False {
            }
            frame True {
              n190 = call "ASYNC_Adam_server.vi"("Values"=w460, "Channel Names"=w459) -> ("Scan Comments"=w457:string[])  [unwired: 1 in, 2 out]
              n191 = Index Array(array=w457, index=0) -> (element=w456:string)
            }
          }
        }
      }
      frame #13 {
        n192 = while {
          tunnel: w464 -> [w478]
          tunnel: w463 -> [w477]
          shift-right: [w465] -> _
          shift-left: _ -> [w472]
          shift-left: _ -> [w471]
          shift-left: _ -> [w470]
          tunnel: [w466] -> w462
          tunnel: [w465] -> w461
          stop <- FALSE continue-if-true
          n193 = call "Read_value_of_earlier_Ch.vi"("Desired Ch to Read"="EnFlo_Lab:Ventilation:Enable", "Ch names"=w477, "Present scan array"=w478) -> ("Value"=w473:dbl, "Scan comment"=w466:string)  [unwired: 1 in]
          n194 = Greater?(x=w473, y=0.5) -> (0:w465:bool)
          n195 = Compound Arithmetic op=AND(w465, w472, invert w471, invert w470) -> (w468:bool)
          n196 = Compound Arithmetic op=AND(invert w465, invert w472, w471, w470) -> (w469:bool)
          n197 = Or(x=w468, y=w469) -> (x .or. y?=w467:bool)
          n198 = case shown="True" w467 {
            tunnel: w473 -> [_ w479]
            frame False {
            }
            frame True {
              n199 = Build Array(1.0 ("element"), w479, w479) -> (w482:dbl[])
              n200 = call "ASYNC_Adam_server.vi"("Values"=w482, "Channel Names"=string[] ["EnFlo_Lab:Window:Enable", "EnFlo_Lab:Window:Open", "EnFlo_Lab:Window_Fans:Enable"]) -> ()  [unwired: 1 in, 3 out]
            }
          }
        }
      }
      frame #14 {
        n201 = while {
          shift-right: [w485] -> _
          shift-left: _ -> [w493]
          shift-left: _ -> [w492]
          shift-left: _ -> [w491]
          tunnel: w484 -> [w486]
          tunnel: w483 -> [w487]
          stop <- FALSE continue-if-true
          # "Opens the West window for ventilation if the EnFlo Tunnel is not measuring"
          n202 = Compound Arithmetic op=AND(w486, invert w487) -> (w485:bool)
          n203 = Compound Arithmetic op=AND(w485, w493, invert w492, invert w491) -> (w489:bool)
          n204 = Compound Arithmetic op=AND(invert w485, invert w493, w492, w491) -> (w490:bool)
          n205 = Or(x=w489, y=w490) -> (x .or. y?=w488:bool)
          n206 = case shown="True" w488 {
            tunnel: w485 -> [_ w495]
            frame False {
            }
            frame True {
              n207 = Select(t=1.0, s=w495, f=0.0) -> (s? t:f=w496:dbl)
              n208 = Build Array(w496, w496) -> (w500:dbl[])
              n209 = call "ASYNC_Adam_server.vi"("Values"=w500, "Channel Names"=string[] ["EnFlo_Lab:West Window:Open1", "EnFlo_Lab:West Window:Open2"]) -> ()  [unwired: 1 in, 3 out]
            }
          }
        }
      }
      frame #15 {
        n210 = while {
          tunnel: w505 -> [w517]
          tunnel: w504 -> [w516]
          shift-right: [w507] -> _
          shift-left: _ -> [w512]
          tunnel: [w511] -> w503
          tunnel: w502 -> [w509]
          tunnel: w501 -> [w506]
          stop <- FALSE continue-if-true
          w508 = "EnFlo_Tunnel:Motor:Enable" ("Desired Ch to Read")
          # "Re Zero EnFlo Tunnel static pressure when turning tunnel on"
          n211 = call "Read_value_of_earlier_Ch.vi"("Desired Ch to Read"=w508, "Ch names"=w516, "Present scan array"=w517) -> ("Value"=w513:dbl, "Scan comment"=w511:string)  [unwired: 1 in]
          n212 = Greater?(x=w513, y=0.5) -> (0:w507:bool)
          n213 = Compound Arithmetic op=AND(w507, invert w512, w506) -> (w510:bool)
          n214 = case shown="False" w510 {
            tunnel: w509 -> [_ w543]
            tunnel: w508 -> [_ w541]
            frame False {
            }
            frame True {
              w540 = "EnFlo_Tunnel:Pressure:Static"
              n215 = To Double Precision Float(number=w543) -> (double precision float=w526:dbl)
              n216 = Build Array(w540) -> (w539:string[])
              n217 = Build Array(w541, w540) -> (w544:string[])
              n218 = Subtract(x=w526, y=15.0) -> (x-y=w524:dbl)
              n219 = call "Get_Current_Scan_server.vi"("Desired Channels"=w539) -> ("Ch Description Array"=w538:T7[])  [unwired: 2 out]
              n220 = Subtract(x=w526, y=3600.0) -> (x-y=w542:dbl)
              n221 = call "Get_ADAM_averages_server.vi"("No of averages"=600, "End time"=w524, "Start time"=w542, "Clients time"=w526, "ADAM Ch Names"=w544) -> ("DBL values"=w528:dbl[][])  [unwired: 1 in, 4 out]
              n222 = Index Array(array=w538) -> (element=w536:T7)  [unwired: 1 in]
              n223 = Unbundle By Name(w536) -> ("A"=w537:dbl)
              n224 = Index Array(array=w528, index (col)=1 ("disabled index (col)")) -> (element=w523:dbl[])  [unwired: 1 in]
              n225 = Index Array(array=w528, index (col)=2 ("disabled index (col)")) -> (element=w522:dbl[])  [unwired: 1 in]
              n226 = Reverse 1D Array(array=w522) -> (reversed array=w518:dbl[])
              n227 = Reverse 1D Array(array=w523) -> (reversed array=w521:dbl[])
              n228 = for {
                tunnel: w521 -> [w546] mode=indexing
                tunnel: [w545] -> w520 mode=indexing
                tunnel: w518 -> [w545] mode=indexing
                stop <- w547 continue-if-true
                n229 = Less?(x=w546, y=0.01) -> (x < y?=w547:bool)
              }
              n230 = call "Mean_fr_NaN_data.vi"("Data"=w520) -> ("Mean value"=w519:dbl)  [unwired: 1 out]
              n231 = Subtract(x=w537, y=w519) -> (x-y=w535:dbl)
              n232 = Bundle By Name(cluster=w536, "A"=w535) -> (w534:T7)
              n233 = Build Array(w534) -> (w533:T7[])
              n234 = call "Update_Ch_Discription_server.vi"("Mode"=T3."Append to Global", "Channels to update In"=w533) -> ()  [unwired: 1 in, 1 out]
            }
          }
        }
      }
      frame #16 {
        # "Resetting A Tunnel speed to zero if the drive in turned off\nso that the belts do not slip when the tunnel is turned on again."
        n235 = while {
          tunnel: w552 -> [w565]
          tunnel: w551 -> [w564]
          shift-right: [w556] -> _
          shift-left: _ -> [w559]
          shift-left: _ -> [w558]
          shift-left: _ -> [w557]
          tunnel: w550 -> [w555]
          tunnel: [w553] -> w549
          stop <- FALSE continue-if-true
          n236 = call "Read_value_of_earlier_Ch.vi"("Desired Ch to Read"="A_Tunnel:Motor:Enable", "Ch names"=w564, "Present scan array"=w565) -> ("Value"=w560:dbl, "Scan comment"=w553:string)  [unwired: 1 in]
          n237 = Less?(x=w560, y=0.5) -> (x < y?=w556:bool)
          n238 = Compound Arithmetic op=AND(w556, w559, invert w558, invert w557, w555) -> (w554:bool)
          n239 = case shown="True" w554 {
            tunnel: w556 -> [_ _]
            frame False {
            }
            frame True {
              w568 = string[] ["A_Tunnel:Speed:Dem Velocity", "A_Tunnel:Speed:Dem Voltage"] ("Channel Names")
              n240 = Array Size(array=w568) -> (size(s)=w569:i32)
              n241 = Initialize Array(0.0 ("element"), w569) -> (w567:dbl[])
              n242 = call "ASYNC_Adam_server.vi"("Values"=w567, "Channel Names"=w568) -> ()  [unwired: 1 in, 3 out]
            }
          }
        }
      }
      frame #17 {
        # "Control Inlet fans"
        n243 = while {
          tunnel: w573 -> [w582]
          tunnel: w572 -> [w583]
          shift-right: [w574] -> _
          shift-left: _ -> [w586]
          tunnel: w571 -> [w588]
          tunnel: [w579] -> w570
          stop <- FALSE continue-if-true
          n244 = call "Read_value_of_earlier_Ch.vi"("Desired Ch to Read"="EnFlo_Tunnel:Reference:Velocity", "Ch names"=w583, "Present scan array"=w582) -> ("Value"=w578:dbl, "Scan comment"=w580:string)  [unwired: 1 in]
          n245 = call "Read_value_of_earlier_Ch.vi"("Desired Ch to Read"="EnFlo_Tunnel:Motor:Enable", "Ch names"=w583, "Present scan array"=w582) -> ("Value"=w589:dbl, "Scan comment"=w581:string)  [unwired: 1 in]
          n246 = Greater?(x=w589, y=0.5) -> (0:w576:bool)
          n247 = Greater?(x=w578, y=0.15) -> (0:w575:bool)
          n248 = And(x=w575, y=w576) -> (x .and. y?=w574:bool)
          n249 = Not Equal?(x=w574, y=w586) -> (x != y?=w585:bool)
          n250 = Compound Arithmetic op=AND(w585, w588) -> (w587:bool)
          n251 = case shown="True" w587 {
            tunnel: w574 -> [_ w594]
            frame False {
            }
            frame True {
              n252 = case shown="True" w594 {
                tunnel: [string[] ["EnFlo_Tunnel:Inlet_Fans:Enable"] ("Channel Names") string[] ["EnFlo_Tunnel:Inlet_Fans:Enable", "Hydrosonic:Transducer:Setting"] ("Channel Names")] -> w596
                tunnel: [1.0 ("element") 0.0 ("element")] -> w593
                frame True {
                }
                frame False {
                }
              }
              n253 = Array Size(array=w596) -> (size(s)=w597:i32)
              n254 = Initialize Array(w593, w597) -> (w595:dbl[])
              n255 = call "ASYNC_Adam_server.vi"("Values"=w595, "Channel Names"=w596) -> ()  [unwired: 1 in, 3 out]
            }
          }
          n256 = Concatenate Strings(w580, w581) -> (w579:string)
        }
      }
      frame #18 {
        # "Control Inlet fans"
        n257 = while {
          tunnel: w605 -> [w616]
          tunnel: w604 -> [w615]
          shift-right: [w606] -> _
          shift-left: _ -> [w607]
          tunnel: w603 -> [w610]
          tunnel: [w608] -> w602
          stop <- FALSE continue-if-true
          n258 = call "Read_value_of_earlier_Ch.vi"("Desired Ch to Read"="LDA:System:Enable", "Ch names"=w615, "Present scan array"=w616) -> ("Value"=w611:dbl, "Scan comment"=w608:string)  [unwired: 1 in]
          n259 = Greater?(x=w611, y=0.5) -> (0:w606:bool)
          n260 = Compound Arithmetic op=AND(w606, invert w607, w610) -> (w609:bool)
          n261 = case shown="True" w609 {
            tunnel: w606 -> [_ _]
            frame False {
            }
            frame True {
              w619 = string[] ["LDA1:Mains_Power:Enable"] ("Channel Names")
              n262 = Array Size(array=w619) -> (size(s)=w620:i32)
              n263 = Initialize Array(1.0 ("element"), w620) -> (w618:dbl[])
              n264 = call "ASYNC_Adam_server.vi"("Values"=w618, "Channel Names"=w619) -> ()  [unwired: 1 in, 3 out]
            }
          }
        }
      }
      frame #19 {
        n265 = And(x=w622, y=w623) -> (x .and. y?=w621:bool)
        n266 = case shown="False" w621 {
          tunnel: w626 -> [w631 _]
          tunnel: w625 -> [w630 _]
          tunnel: [w627 ""] -> w624
          frame False {
            n267 = for {
              tunnel: w631 -> [w641]
              tunnel: w630 -> [w640]
              tunnel: string[] ["EnFlo_Tunnel:Heater:Enable", "EnFlo_Tunnel:Chiller_Pump:Enable", "EnFlo_Tunnel:Tap_Water:Enable"] ("Ch Names") -> [w636] mode=indexing
              shift-right: [w634] -> w627
              shift-left: "" -> [w635]
              n268 = call "Read_value_of_earlier_Ch.vi"("Desired Ch to Read"=w636, "Ch names"=w640, "Present scan array"=w641) -> ("Value"=w638:dbl, "Scan comment"=w633:string)  [unwired: 1 in]
              n269 = Greater?(x=w638, y=0.5) -> (0:w637:bool)
              n270 = case shown="True" w637 {
                tunnel: w636 -> [_ w646]
                tunnel: ["" w643] -> w632
                frame False {
                }
                frame True {
                  n271 = Build Array(w646) -> (w649:string[])
                  n272 = Build Array(0.0) -> (w648:dbl[])
                  n273 = call "ASYNC_Adam_server.vi"("Values"=w648, "Channel Names"=w649) -> ("Scan Comments"=w644:string[])  [unwired: 1 in, 2 out]
                  n274 = Index Array(array=w644, index=0) -> (element=w643:string)
                }
              }
              n275 = Concatenate Strings(w635, w633, w632) -> (w634:string)
            }
          }
          frame True {
          }
        }
      }
      frame #20 {
        n276 = call "Read_value_of_earlier_Ch.vi"("Desired Ch to Read"="EnFlo_Tunnel:Reference:Velocity", "Ch names"=w656, "Present scan array"=w657) -> ("Value"=w659:dbl, "Scan comment"=w653:string)  [unwired: 1 in]
        n277 = Less?(x=w659, y=0.25) -> (x < y?=w658:bool)
        n278 = And(x=w651, y=w658) -> (x .and. y?=w655:bool)
        n279 = case shown="True" w655 {
          tunnel: ["" w664] -> w654
          frame False {
          }
          frame True {
            n280 = Build Array("EnFlo_Tunnel:Heater:Enable") -> (w669:string[])
            n281 = Build Array(0.0) -> (w668:dbl[])
            n282 = call "ASYNC_Adam_server.vi"("Values"=w668, "Channel Names"=w669) -> ("Scan Comments"=w665:string[])  [unwired: 1 in, 2 out]
            n283 = Index Array(array=w665, index=0) -> (element=w664:string)
          }
        }
        n284 = Concatenate Strings(w653, w654) -> (w652:string)
      }
      frame #21 {
        w671 = "EnFlo_Tunnel:Chiller_Pump_2:Dem_Power(%)" ("Ch Name")
        n285 = case shown="True" w672 {
          tunnel: w677 -> [_ w687]
          tunnel: w676 -> [_ w686]
          tunnel: [FALSE w684] -> w675
          tunnel: ["" w680] -> w673
          tunnel: w671 -> [_ w683]
          frame False {
          }
          frame True {
            n286 = call "Read_value_of_earlier_Ch.vi"("Desired Ch to Read"=w683, "Ch names"=w686, "Present scan array"=w687) -> ("Value"=w692:dbl, "Scan comment"=w682:string)  [unwired: 1 in]
            n287 = call "Read_value_of_earlier_Ch.vi"("Desired Ch to Read"="EnFlo_Tunnel:Floor_Cooling:Enable", "Ch names"=w686, "Present scan array"=w687) -> ("Value"=w689:dbl, "Scan comment"=w681:string)  [unwired: 1 in]
            n288 = Concatenate Strings(w682, w681) -> (w680:string)
            n289 = Greater?(x=w692, y=0.5) -> (0:w685:bool)
            n290 = Less?(x=w689, y=0.5) -> (x < y?=w688:bool)
            n291 = And(x=w685, y=w688) -> (x .and. y?=w684:bool)
          }
        }
        n292 = case shown="True" w675 {
          tunnel: ["" w696] -> w674
          tunnel: w671 -> [_ w695]
          frame False {
          }
          frame True {
            n293 = Build Array(0.0) -> (w700:dbl[])
            n294 = Build Array(w695) -> (w701:string[])
            n295 = call "ASYNC_Adam_server.vi"("Values"=w700, "Channel Names"=w701) -> ("Scan Comments"=w697:string[])  [unwired: 1 in, 2 out]
            n296 = Index Array(array=w697, index=0) -> (element=w696:string)
          }
        }
        n297 = Concatenate Strings(w673, w674) -> (w670:string)
      }
      frame #22 {
        n298 = call "Read_Earlier_Channels.vi"("Present scan array"=w708, "Ch names"=w709, "Desired Channels"=string[] ["Tank:Fill:Now", "Tank:Desired_Depth:mm", "Tank:Depth:mm", "Tank:Fill_Valve:Enable"]) -> ("Scan comments"=w716:string, "Index 0"=w722:dbl, "Index 1"=w719:dbl, "Index 2"=w718:dbl, "Index 3"=w720:dbl)  [unwired: 1 out]
        n299 = call "Read_value_of_earlier_Ch.vi"("Desired Ch to Read"="EnFlo Lab:Leak_Detector:Happy", "Ch names"=w709, "Present scan array"=w708) -> ("Value"=w706:dbl, "Scan comment"=w702:string)  [unwired: 1 in]
        n300 = Greater?(x=w722, y=0.5) -> (0:w705:bool)
        n301 = Greater?(x=w720, y=0.5) -> (0:w717:bool)
        n302 = Greater?(x=w706, y=0.5) -> (0:w703:bool)
        n303 = And(x=w703, y=w705) -> (x .and. y?=w704:bool)
        n304 = case shown="False" w704 {
          tunnel: w719 -> [_ w737]
          tunnel: w718 -> [_ w736]
          tunnel: w717 -> [w725 w732]
          tunnel: [w726 w734] -> w712
          tunnel: [w727 w733] -> w711
          frame False {
            n305 = case shown="True" w725 {
              tunnel: [dbl[] [] ("appended array") dbl[] [0.0] ("appended array")] -> w727
              tunnel: [string[] [] ("Desired Channels") string[] ["Tank:Fill_Valve:Enable"] ("Desired Channels")] -> w726
              frame False {
              }
              frame True {
                (unwired) "Tank:Fill_Valve:Enable"
              }
            }
          }
          frame True {
            n306 = Greater?(x=w737, y=w736) -> (0:w735:bool)
            n307 = case shown="True" w735 {
              tunnel: [string[] ["Tank:Fill:Now", "Tank:Fill_Valve:Enable"] ("Desired Channels") w742] -> w734
              tunnel: [dbl[] [0.0, 0.0] ("appended array") w741] -> w733
              tunnel: w732 -> [_ w740]
              frame False {
              }
              frame True {
                n308 = case shown="True" w740 {
                  tunnel: [string[] ["Tank:Fill_Valve:Enable"] ("Desired Channels") string[] [] ("Desired Channels")] -> w742
                  tunnel: [dbl[] [1.0] ("appended array") dbl[] [] ("appended array")] -> w741
                  frame False {
                    (unwired) "Tank:Fill_Valve:Enable"
                  }
                  frame True {
                  }
                }
              }
            }
          }
        }
        n309 = call "ASYNC_Adam_server.vi"("Values"=w711, "Channel Names"=w712) -> ("Scan Comments"=w713:string[])  [unwired: 1 in, 2 out]
        n310 = Concatenate Strings(w713) -> (w714:string)
        n311 = Concatenate Strings(w702, w714, w716) -> (w715:string)
      }
      frame #23 {
        n312 = call "Read_value_of_earlier_Ch.vi"("Desired Ch to Read"="EnFlo_Tunnel:Reference:Velocity", "Ch names"=w751, "Present scan array"=w752) -> ("Value"=w749:dbl, "Scan comment"=w747:string)  [unwired: 1 in]
        n313 = Greater?(x=w749, y=0.4) -> (0:w755:bool)
        n314 = Compound Arithmetic op=AND(w748, w755) -> (w753:bool)
      }
      frame #24 {
        w764 = "EnFlo_Tunnel:Heat_Ex_Div_Valve:Dem Pos"
        n315 = case shown="True" w765 {
          tunnel: w767 -> [_ w802]
          tunnel: w766 -> [_ w803]
          tunnel: w764 -> [_ w806]
          tunnel: [0.0 ("upper limit") w812] -> w762
          tunnel: ["" w797] -> w759
          frame False {
          }
          frame True {
            n316 = call "Read_value_of_earlier_Ch.vi"("Desired Ch to Read"="EnFlo_Tunnel:Exit Duct:Dem Temp", "Ch names"=w803, "Present scan array"=w802) -> ("Value"=w811:dbl, "Scan comment"=w801:string)  [unwired: 1 in]
            n317 = call "Read_value_of_earlier_Ch.vi"("Desired Ch to Read"="EnFlo_Tunnel:Exit Duct Top:Temp", "Ch names"=w803, "Present scan array"=w802) -> ("Value"=w807:dbl, "Scan comment"=w800:string)  [unwired: 1 in]
            n318 = call "Read_value_of_earlier_Ch.vi"("Desired Ch to Read"="EnFlo_Tunnel:Exit Duct:Temp", "Ch names"=w803, "Present scan array"=w802) -> ("Value"=w808:dbl, "Scan comment"=w799:string)  [unwired: 1 in]
            n319 = call "Read_value_of_earlier_Ch.vi"("Desired Ch to Read"=w806, "Ch names"=w803, "Present scan array"=w802) -> ("Value"=w809:dbl, "Scan comment"=w798:string)  [unwired: 1 in]
            n320 = Add(x=w807, y=w808) -> (x+y=w816:dbl)
            n321 = Divide(x=w816, y=2.0) -> (x/y=w818:dbl)
            n322 = Concatenate Strings(w801, w800, w799, w798) -> (w797:string)
            n323 = call "Back_End_Chiller_PID.vi"("Present Value"=w818, "Previous Control Sum"=w809, "Setpoint"=w811) -> ("Dem Output"=w815:dbl)
            n324 = In Range and Coerce(upper limit=100.0, x=w815, lower limit=0.0) -> (coerced(x)=w812:dbl)  [unwired: 1 out]
          }
        }
        n325 = case shown="False" w756 {
          tunnel: [w769 w780] -> w763
          tunnel: w762 -> [_ w780]
          tunnel: [w768 FALSE] -> w760
          frame False {
            # "Exercise valve once a week"
            n326 = Seconds To Date/Time() -> (date time rec=w770:T5)  [unwired: 2 out]
            n327 = Unbundle By Name(w770) -> ("day of week"=w775:i32, "hour"=w773:i32)
            n328 = Less?(x=w773, y=3) -> (x < y?=w778:bool)
            n329 = Equal?(x=7, y=w775) -> (x = y?=w777:bool)
            n330 = And(x=w777, y=w778) -> (x .and. y?=w768:bool)
            n331 = Select(t=100.0, s=w768, f=0.0) -> (s? t:f=w769:dbl)
          }
          frame True {
          }
        }
        n332 = while {
          shift-right: [w786] -> _
          shift-left: _ -> [w787]
          tunnel: w763 -> [w786]
          tunnel: w764 -> [w788]
          tunnel: w761 -> [w783]
          tunnel: [w781] -> w758
          stop <- TRUE stop-if-true
          n333 = Not Equal?(x=w786, y=w787) -> (x != y?=w784:bool)
          n334 = Compound Arithmetic op=OR(w784, invert w783) -> (w782:bool)
          n335 = Build Array(w788) -> (w789:string[])
          n336 = Build Array(w786) -> (w790:dbl[])
          n337 = case shown="True" w782 {
            tunnel: w790 -> [_ w794]
            tunnel: w789 -> [_ w793]
            tunnel: [string[] [] ("Scan Comments") w792] -> w781
            frame False {
            }
            frame True {
              n338 = call "ASYNC_Adam_server.vi"("Values"=w794, "Channel Names"=w793) -> ("Scan Comments"=w792:string[])  [unwired: 1 in, 2 out]
            }
          }
        }
        n339 = Concatenate Strings(w759, w758) -> (w757:string)
      }
      frame #25 {
        n340 = while {
          shift-right: [w826] -> _
          shift-left: _ -> [w827]
          tunnel: w821 -> [w826]
          tunnel: [w823] -> w820
          tunnel: w819 -> [w822]
          stop <- TRUE stop-if-true
          n341 = Compound Arithmetic op=AND(w822, invert w827, w826) -> (w824:bool)
          n342 = case shown="True" w824 {
            tunnel: ["" w830] -> w823
            frame False {
            }
            frame True {
              n343 = Build Array("EnFlo Lab:Heat:Extraction") -> (w835:string[])
              n344 = Build Array(0.0) -> (w834:dbl[])
              n345 = call "ASYNC_Adam_server.vi"("Values"=w834, "Channel Names"=w835) -> ("Scan Comments"=w831:string[])  [unwired: 1 in, 2 out]
              n346 = Index Array(array=w831, index=0) -> (element=w830:string)
            }
          }
        }
      }
      frame #26 {
        # "To automatically control the request for the University Stall chiller to run."
        n347 = while {
          tunnel: w840 -> [w848]
          tunnel: w839 -> [w849]
          shift-right: [w843] -> _
          shift-left: _ -> [w858]
          shift-left: _ -> [w857]
          shift-left: _ -> [w856]
          tunnel: [w842] -> w838
          tunnel: [w841] -> w837
          stop <- FALSE continue-if-true
          n348 = Build Array("EnFlo_Tunnel:Chiller_Pump:Enable" ("Desired Ch to Read"), "Aero_Tunnel:Cooling_Pump:Enable" ("Desired Ch to Read")) -> (w850:string[])
          n349 = call "Read_Earlier_Channels.vi"("Present scan array"=w848, "Ch names"=w849, "Desired Channels"=w850) -> ("Scan comments"=w841:string, "Index 0"=w847:dbl, "Index 1"=w846:dbl)  [unwired: 3 out]
          n350 = Build Array(w847, w846) -> (w845:dbl[])
          n351 = Greater?(x=w845, y=0.5) -> (0:w844:bool[])
          n352 = Or Array Elements(Boolean array=w844) -> (logical OR=w843:bool)
          n353 = Compound Arithmetic op=AND(w843, w858, invert w857, invert w856) -> (w854:bool)
          n354 = Compound Arithmetic op=AND(invert w843, invert w858, w857, w856) -> (w855:bool)
          n355 = Or(x=w854, y=w855) -> (x .or. y?=w853:bool)
          n356 = case shown="True" w853 {
            tunnel: w843 -> [_ w867]
            tunnel: [string[] [] ("Scan Comments") w862] -> w842
            frame False {
            }
            frame True {
              n357 = case shown="False" w867 {
                tunnel: [string[] ["University:Chilled Water:Requested"] ("Channel Names") string[] ["University:Chilled Water:Requested"] ("Channel Names")] -> w866
                tunnel: [1.0 ("y") 0.0 ("y")] -> w863
                frame True {
                }
                frame False {
                }
              }
              n358 = Array Size(array=w866) -> (size(s)=w864:i32)
              n359 = Initialize Array(w863, w864) -> (w865:dbl[])
              n360 = call "ASYNC_Adam_server.vi"("Values"=w865, "Channel Names"=w866) -> ("Scan Comments"=w862:string[])  [unwired: 1 in, 2 out]
            }
          }
        }
        n361 = Concatenate Strings(w838, w837) -> (w836:string)
      }
      frame #27 {
        # "Exercise the floor cooling valve once a week"
        n362 = while {
          shift-right: [w876] -> _
          shift-left: _ -> [w881]
          tunnel: w874 -> [w876]
          tunnel: w873 -> [w878]
          tunnel: [w875] -> w872
          stop <- TRUE stop-if-true
          n363 = Not Equal?(x=w876, y=w881) -> (x != y?=w879:bool)
          n364 = Compound Arithmetic op=AND(w879, w878) -> (w877:bool)
          n365 = case shown="True" w877 {
            tunnel: w876 -> [_ w888]
            tunnel: ["" w883] -> w875
            frame False {
            }
            frame True {
              n366 = Select(t=1.0, s=w888, f=0.0) -> (s? t:f=w889:dbl)
              n367 = Build Array(w889) -> (w892:dbl[])
              n368 = Build Array("EnFlo_Tunnel:Floor_Cooling:Enable") -> (w891:string[])
              n369 = call "ASYNC_Adam_server.vi"("Values"=w892, "Channel Names"=w891) -> ("Scan Comments"=w884:string[])  [unwired: 1 in, 2 out]
              n370 = Index Array(array=w884, index=0) -> (element=w883:string)
            }
          }
        }
      }
      frame #28 {
        n371 = Build Array("GMU:CO2_Low:Siren") -> (w893:string[])
        n372 = Quotient & Remainder(x=w907, y=15) -> (x-y*floor(x/y)=w905:i32)  [unwired: 1 out]
        n373 = call "Get_Current_Scan_server.vi"("Desired Channels"=w893) -> ("Ch Description Array"=w911:T7[], "Numerical Values"=w901:dbl[])  [unwired: 1 out]
        n374 = Equal To 0?(x=w905) -> (x = 0?=w904:bool)
        n375 = Select(t=1.0, s=w904, f=0.0) -> (s? t:f=w903:dbl)
        n376 = Index Array(array=w911, index=0) -> (element=w910:T7)
        n377 = Index Array(array=w901, index=0) -> (element=w898:dbl)
        n378 = Unbundle By Name(w910) -> ("A"=w909:dbl)
        n379 = Greater?(x=w898, y=0.5) -> (0:w896:bool)
        n380 = Greater?(x=w909, y=0.5) -> (0:w897:bool)
        n381 = Or(x=w897, y=w896) -> (x .or. y?=w895:bool)
        n382 = while {
          shift-right: [w921] -> _
          shift-left: _ -> [w922]
          tunnel: w903 -> [w921]
          tunnel: [w917] -> w894
          tunnel: w895 -> [w916]
          tunnel: w893 -> [w915]
          stop <- TRUE stop-if-true
          n383 = Not Equal?(x=w921, y=w922) -> (x != y?=w919:bool)
          n384 = Build Array(w921) -> (w923:dbl[])
          n385 = Compound Arithmetic op=AND(w919, w916) -> (w918:bool)
          n386 = case shown="True" w918 {
            tunnel: w923 -> [_ w929]
            tunnel: w915 -> [_ w928]
            tunnel: ["" w925] -> w917
            frame False {
            }
            frame True {
              n387 = call "ASYNC_Adam_server.vi"("Values"=w929, "Channel Names"=w928) -> ("Scan Comments"=w926:string[])  [unwired: 1 in, 2 out]
              n388 = Index Array(array=w926, index=0) -> (element=w925:string)
            }
          }
        }
      }
      frame #29 {
        n389 = Concatenate Strings(w930, w931, w933, w932, w934, w935, w936, w937, w938, w944, w945, w946, w947, w948, w949, w950, w957, w956, w955, w954, w953, w952, w951, w942, w941, w940, w939) -> (→"Scan comment":string)
      }
    }
  }
